vi "Create.vi"(8 "error in (no error)":errorcluster, 10 "messageID":u16) -> (0 "error out":errorcluster, 3 "mqttCmdPublishReceived out":refnum<class "PublishReceivedMqttMsg.lvclass">)   [LabVIEW 2020, in "PublishReceivedMqttMsg.lvclass"]
uses:
  PublishReceivedMqttMsg.lvclass
  PublishReceivedMqttMsg.lvclass/PublishReceivedMqttMsg.ctl
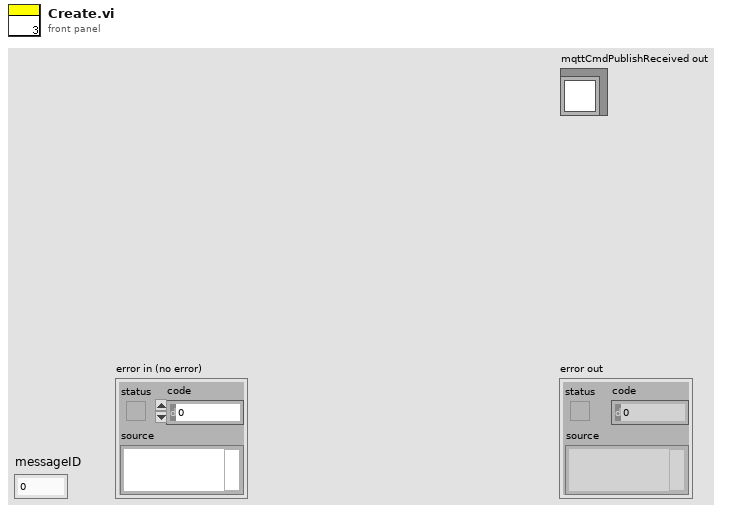
[diagram p1: front panel]
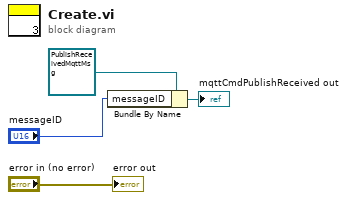
[diagram p0: block diagram]
diagram:
  n1 = Bundle By Name(cluster=refnum<class "PublishReceivedMqttMsg.lvclass"> refnum ("mqttCmdPublishReceived in"), "messageID"="messageID") -> (→"mqttCmdPublishReceived out":refnum<class "PublishReceivedMqttMsg.lvclass">)
  "error out" <- "error in (no error)"
